vi "AddNewProtocolEntry.vi"(11 "Array (Eingang)":refnum<vi>) -> (0 "Fehler (Ausgang)":errorcluster, 3 "Referenz (Ausgang)":refnum<vi>)   [LabVIEW 2014]
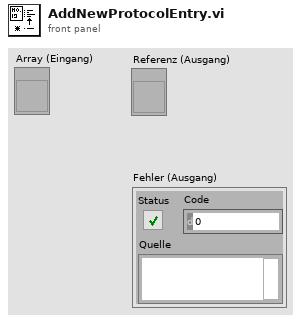
[diagram p1: front panel]
types:
  T1 = typedef "ProtocolT.ctl" = T2[]
  T2 = typedef "ProtocolEntry.ctl" = cluster{"Zeitstempel":timestamp, "String":string, "Abbrechen-Schaltfläche":bool, "Optionen-Schaltfläche":bool}
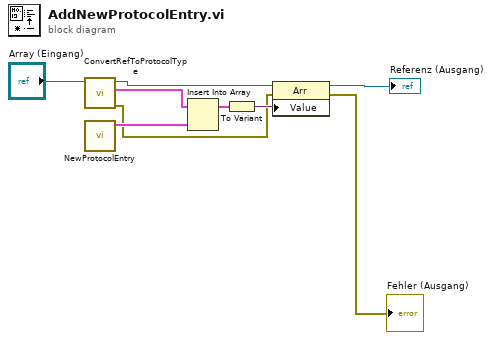
[diagram p0: block diagram]
diagram:
  n1 = call "ConvertRefToProtocolType.vi"("Array (Eingang)"="Array (Eingang)") -> ("Fehler (Ausgang)"=w4:errorcluster, "ProtocolT"=w7:T1, "Array (Ausgang)"=w3:refnum<vi>)  [unwired: 8 in]
  n2 = call "NewProtocolEntry.vi"() -> ("ProtocolEntryT 2"=w6:T2)  [unwired: 11 in]
  n3 = Insert Into Array(array=w7, new element=w6) -> (w8:T1)  [unwired: 1 in]
  n4 = To Variant(anything=w8) -> (Variant=w9:variant)
  n5 = property class="Arr"(reference=w3, error in=w4, "Value"=w9) -> (reference out=→"Referenz (Ausgang)":refnum<vi>, error out=→"Fehler (Ausgang)":errorcluster)
